vi "Sub_predictor_v4(SubVI).vi"(6 "predicted step":dbl=0.04 format="%#_13g", 8 "Sim_running":bool, 9 "q_i":dbl[](array[numeric]), 10 "Pred ?":bool, 11 "t [s]":dbl) -> (0 "Euler Angles Table [deg]":dbl[](array[numeric]), 1 "Elevation/Azimuth [deg]":dbl[](array[numeric]), 3 "Euler Angles Table_pred [deg]":dbl[](array[numeric]), 4 "DMARS SIM pred [º]":cluster{"phi":dbl, "theta":dbl, "psi":dbl})   [LabVIEW 2017]
uses:
  <vilib>/Analysis/coordinate.llb/Euler Rotation Order.ctl
  <vilib>/Analysis/_algsub.llb/Real PseudoInverse Matrix.vi
  <vilib>/Analysis/baseanly.llb/Real A x B.vi
  <vilib>/Analysis/Matrix/Numeric/Conversions/Array To Matrix - RA2.vi
  <vilib>/Analysis/Matrix/Numeric/Conversions/Array To Matrix - RA.vi
  <vilib>/Analysis/Matrix/Numeric/Conversions/Matrix To Array - RM.vi
  <vilib>/Analysis/Matrix/NI_Matrix.lvlib
  <vilib>/Analysis/NI_AALPro.lvlib
  <vilib>/Analysis/NI_AALBase.lvlib
  <vilib>/Analysis/7linalg.llb/Real Transpose Matrix.vi
panel:
  out "DCM":dbl[][](array[numeric])
  out "Elevation [deg]":dbl
  out "Azimuth [deg]":dbl
  in  "Euler Angles [º] debug":cluster{"phi":dbl, "theta":dbl, "psi":dbl}
  out "Azimuth [rad]":dbl
  out "Elevation [rad]":dbl
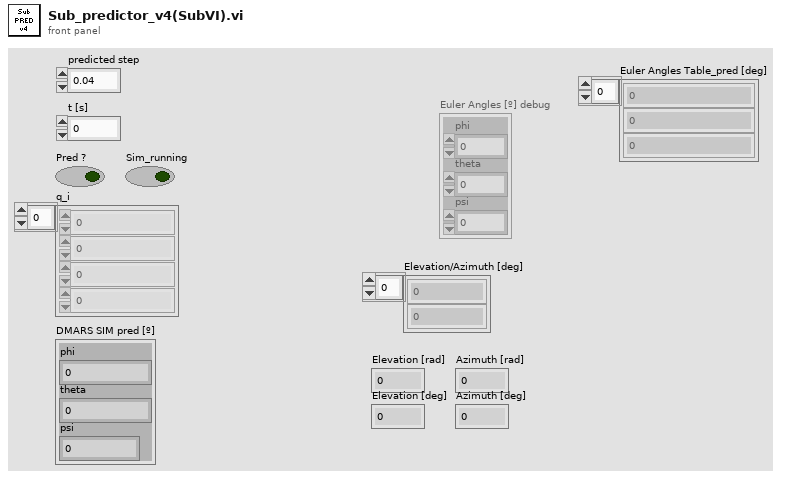
[diagram p1: front panel]
types:
  T1 = typedef "NI_Matrix.lvlib/RealMatrix.ctl" = dbl[][]
  T2 = typedef "NI_AALPro.lvlib/Euler Rotation Order.ctl" = u16
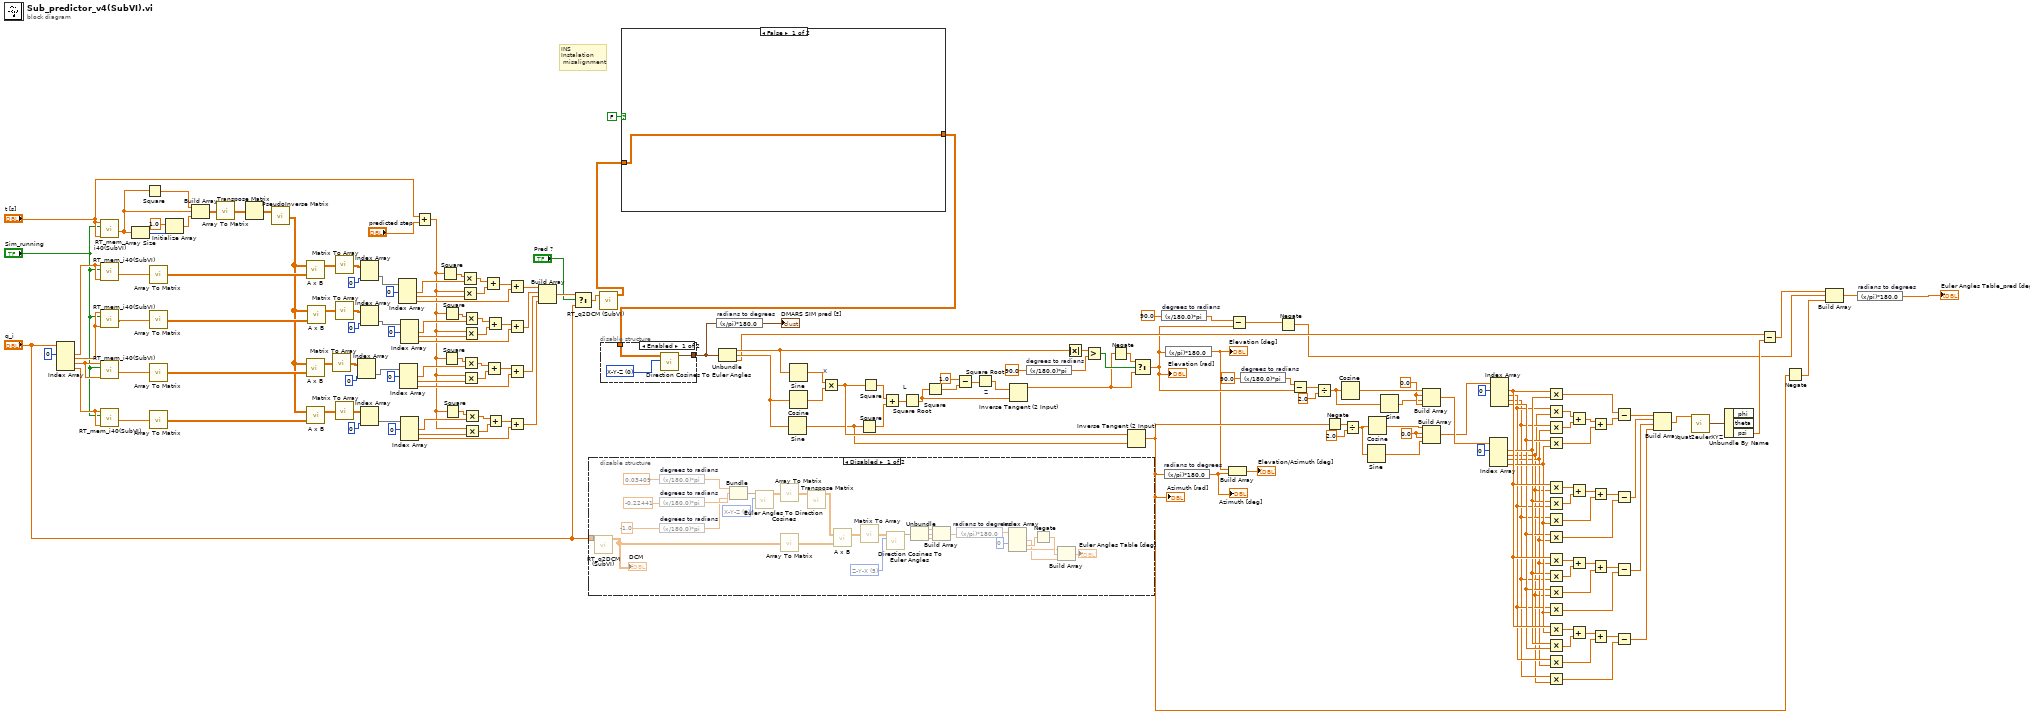
[diagram p0: block diagram]
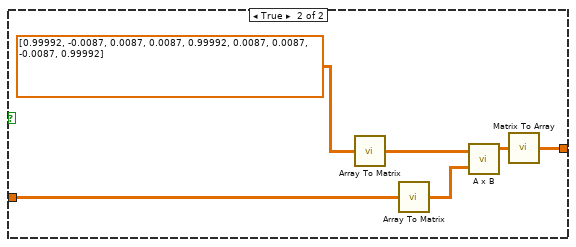
[diagram p2: hidden frame]
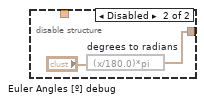
[diagram p4: hidden frame]
diagram:
  w72 = 0.0 ("element")
  w79 = 0.0 ("element")
  # "INS\nInstalation\n misalignment"
  n1 = Index Array(array="q_i", index #1=0 ("index")) -> (element #1=w101:dbl, element #2=w106:dbl, element #3=w107:dbl, element #4=w108:dbl)  [unwired: 3 in]
  n2 = call "RT_mem_i40(SubVI).vi"("Ini_val"="t [s]", "start"="Sim_running", "In"="t [s]") -> ("output array"=w109:dbl[])  [unwired: 8 in]
  n3 = call "RT_mem_i40(SubVI).vi"("Ini_val"=w101, "start"="Sim_running", "In"=w101) -> ("output array"=w104:dbl[])  [unwired: 8 in]
  n4 = call "RT_mem_i40(SubVI).vi"("Ini_val"=w106, "start"="Sim_running", "In"=w106) -> ("output array"=w105:dbl[])  [unwired: 8 in]
  n5 = call "RT_mem_i40(SubVI).vi"("Ini_val"=w107, "start"="Sim_running", "In"=w107) -> ("output array"=w103:dbl[])  [unwired: 8 in]
  n6 = call "RT_mem_i40(SubVI).vi"("Ini_val"=w108, "start"="Sim_running", "In"=w108) -> ("output array"=w102:dbl[])  [unwired: 8 in]
  n7 = Array Size(array=w109) -> (size(s)=w160:i32)
  n8 = Square(x=w109) -> (x^2=w162:dbl[])
  n9 = call-poly <vilib>:"Array To Matrix.vi"("Real 1D Array"=w104) -> ("Real Matrix (Column Vector)"=w171:T1)
  n10 = call-poly <vilib>:"Array To Matrix.vi"("Real 1D Array"=w105) -> ("Real Matrix (Column Vector)"=w167:T1)
  n11 = call-poly <vilib>:"Array To Matrix.vi"("Real 1D Array"=w103) -> ("Real Matrix (Column Vector)"=w172:T1)
  n12 = call-poly <vilib>:"Array To Matrix.vi"("Real 1D Array"=w102) -> ("Real Matrix (Column Vector)"=w159:T1)
  n13 = Initialize Array(1.0 ("element"), w160) -> (w163:dbl[])
  n14 = Build Array(w162, w109, w163) -> (w165:dbl[][])
  n15 = call-poly <vilib>:"Array To Matrix.vi"("Real 2D Array"=w165) -> ("Real Matrix"=w164:T1)
  n16 = Transpose Matrix(1:w164) -> (0:w166:T1)
  n17 = call-poly <vilib>:"PseudoInverse Matrix.vi"("Input Matrix"=w166) -> ("PseudoInverse Matrix"=w155:T1)  [unwired: 1 in, 1 out]
  n18 = call-poly <vilib>:"A x B.vi"("B"=w171, "A"=w155) -> ("A x B"=w177:T1)  [unwired: 1 out]
  n19 = call-poly <vilib>:"A x B.vi"("B"=w172, "A"=w155) -> ("A x B"=w178:T1)  [unwired: 1 out]
  n20 = call-poly <vilib>:"A x B.vi"("B"=w159, "A"=w155) -> ("A x B"=w156:T1)  [unwired: 1 out]
  n21 = call-poly <vilib>:"A x B.vi"("B"=w167, "A"=w155) -> ("A x B"=w170:T1)  [unwired: 1 out]
  n22 = call-poly <vilib>:"Matrix To Array.vi"("Real Matrix"=w178) -> ("Real 2D Array"=w175:dbl[][])
  n23 = call-poly <vilib>:"Matrix To Array.vi"("Real Matrix"=w177) -> ("Real 2D Array"=w174:dbl[][])
  n24 = call-poly <vilib>:"Matrix To Array.vi"("Real Matrix"=w170) -> ("Real 2D Array"=w168:dbl[][])
  n25 = call-poly <vilib>:"Matrix To Array.vi"("Real Matrix"=w156) -> ("Real 2D Array"=w158:dbl[][])
  n26 = Index Array(array=w175, index (col)=0 ("index (row)")) -> (element=w118:dbl[])  [unwired: 1 in]
  n27 = Index Array(array=w174, index (col)=0 ("index (row)")) -> (element=w144:dbl[])  [unwired: 1 in]
  n28 = Index Array(array=w168, index (col)=0 ("index (row)")) -> (element=w119:dbl[])  [unwired: 1 in]
  n29 = Index Array(array=w158, index (col)=0 ("index (row)")) -> (element=w117:dbl[])  [unwired: 1 in]
  n30 = Index Array(array=w144, index #1=0 ("index")) -> (element #1=w147:dbl, element #2=w149:dbl, element #3=w152:dbl)  [unwired: 2 in]
  n31 = Index Array(array=w118, index #1=0 ("index")) -> (element #1=w130:dbl, element #2=w132:dbl, element #3=w135:dbl)  [unwired: 2 in]
  n32 = Index Array(array=w119, index #1=0 ("index")) -> (element #1=w141:dbl, element #2=w139:dbl, element #3=w136:dbl)  [unwired: 2 in]
  n33 = Index Array(array=w117, index #1=0 ("index")) -> (element #1=w125:dbl, element #2=w123:dbl, element #3=w120:dbl)  [unwired: 2 in]
  n34 = Add(x="t [s]", y="predicted step") -> (x+y=w116:dbl)
  n35 = Square(x=w116) -> (x^2=w146:dbl)
  n36 = Square(x=w116) -> (x^2=w129:dbl)
  n37 = Square(x=w116) -> (x^2=w142:dbl)
  n38 = Square(x=w116) -> (x^2=w126:dbl)
  n39 = Multiply(x=w146, y=w147) -> (x*y=w148:dbl)
  n40 = Multiply(x=w116, y=w149) -> (x*y=w150:dbl)
  n41 = Multiply(x=w129, y=w130) -> (x*y=w131:dbl)
  n42 = Multiply(x=w116, y=w132) -> (x*y=w133:dbl)
  n43 = Multiply(x=w142, y=w141) -> (x*y=w140:dbl)
  n44 = Multiply(x=w116, y=w139) -> (x*y=w138:dbl)
  n45 = Multiply(x=w126, y=w125) -> (x*y=w124:dbl)
  n46 = Multiply(x=w116, y=w123) -> (x*y=w122:dbl)
  n47 = Add(x=w148, y=w150) -> (x+y=w151:dbl)
  n48 = Add(x=w131, y=w133) -> (x+y=w134:dbl)
  n49 = Add(x=w140, y=w138) -> (x+y=w137:dbl)
  n50 = Add(x=w124, y=w122) -> (x+y=w121:dbl)
  n51 = Add(x=w151, y=w152) -> (x+y=w115:dbl)
  n52 = Add(x=w137, y=w136) -> (x+y=w114:dbl)
  n53 = Add(x=w134, y=w135) -> (x+y=w113:dbl)
  n54 = Add(x=w121, y=w120) -> (x+y=w112:dbl)
  n55 = Build Array(w115, w114, w113, w112) -> (w8:dbl[])
  n56 = Select(t=w8, s="Pred ?", f="q_i") -> (s? t:f=w7:dbl[])
  n57 = disable-structure shown="Disabled" {
    disable-tunnel: "q_i" -> [w206 _]
    frame Disabled {
      w191 = T2 0 items=["X-Y-Z", "X-Z-Y", "Y-X-Z", "Y-Z-X", "Z-X-Y", "Z-Y-X", "X-Y-X", "X-Z-X", "Y-X-Y", "Y-Z-Y", "Z-X-Z", "Z-Y-Z"] ("rotation order")
      w193 = T2 5 items=["X-Y-Z", "X-Z-Y", "Y-X-Z", "Y-Z-X", "Z-X-Y", "Z-Y-X", "X-Y-X", "X-Z-X", "Y-X-Y", "Y-Z-Y", "Z-X-Z", "Z-Y-Z"] ("rotation order")
      n58 = call "RT_q2DCM (SubVI).vi"("Quaternion"=w206) -> ("DCM"=w207:dbl[][])  [unwired: 10 in]
      "DCM" <- w207
      n59 = expression code="(x/180.0)*pi" "degrees to radians"(0.03409 ("y")) -> (w190:dbl)
      n60 = expression code="(x/180.0)*pi" "degrees to radians"(-0.22441 ("y")) -> (w189:dbl)
      n61 = expression code="(x/180.0)*pi" "degrees to radians"(-1.0 ("y")) -> (w188:dbl)
      n62 = Bundle("y"=w190, "y"=w189, "y"=w188) -> (w192:cluster{"y":dbl, "y":dbl, "y":dbl})  [unwired: 1 in]
      n63 = call <vilib>:"Euler Angles To Direction Cosines.vi"("rotation order"=w191, "Euler Angles"=w192) -> ("Direction Cosines"=w185:dbl[][])  [unwired: 8 in, 1 out]
      n64 = call-poly <vilib>:"Array To Matrix.vi"("Real 2D Array"=w185) -> ("Real Matrix"=w184:T1)
      n65 = call-poly <vilib>:"Array To Matrix.vi"("Real 2D Array"=w207) -> ("Real Matrix"=w183:T1)
      n66 = call-poly <vilib>:"Transpose Matrix.vi"("Input Matrix"=w184) -> ("Matrix Transpose"=w182:T1)  [unwired: 9 in, 1 out]
      n67 = call-poly <vilib>:"A x B.vi"("B"=w183, "A"=w182) -> ("A x B"=w181:T1)  [unwired: 1 out]
      n68 = call-poly <vilib>:"Matrix To Array.vi"("Real Matrix"=w181) -> ("Real 2D Array"=w180:dbl[][])
      n69 = call <vilib>:"Direction Cosines To Euler Angles.vi"("rotation order"=w193, "Direction Cosines"=w180) -> ("Euler Angles"=w196:cluster{"phi":dbl, "theta":dbl, "psi":dbl})  [unwired: 8 in, 1 out]
      n70 = Unbundle(w196) -> ("phi"=w194:dbl, "theta"=w195:dbl, "psi"=w197:dbl)
      n71 = Build Array(w194, w195, w197) -> (w205:dbl[])
      n72 = expression code="(x/pi)*180.0" "radians to degrees"(w205) -> (w201:dbl[])
      n73 = Index Array(array=w201, index #1=0 ("index")) -> (element #1=w199:dbl, element #2=w204:dbl, element #3=w202:dbl)  [unwired: 2 in]
      n74 = Negate(x=w204) -> (-x=w203:dbl)
      n75 = Build Array(w202, w203, w199) -> (→"Euler Angles Table [deg]":dbl[])
    }
    frame Enabled {
    }
  }
  n76 = call "RT_q2DCM (SubVI).vi"("Quaternion"=w7) -> ("DCM"=w3:dbl[][])  [unwired: 10 in]
  n77 = case shown="False" FALSE {
    tunnel: [w208 w211] -> w2
    tunnel: w3 -> [w208 w209]
    frame False {
    }
    frame True {
      n78 = call-poly <vilib>:"Array To Matrix.vi"("Real 2D Array"=dbl[][] [[0.99992, -0.0087, 0.0087], [0.0087, 0.99992, 0.0087], [0.0087, -0.0087, 0.99992]]) -> ("Real Matrix"=w213:T1)
      n79 = call-poly <vilib>:"Array To Matrix.vi"("Real 2D Array"=w209) -> ("Real Matrix"=w212:T1)
      n80 = call-poly <vilib>:"A x B.vi"("B"=w212, "A"=w213) -> ("A x B"=w214:T1)  [unwired: 1 out]
      n81 = call-poly <vilib>:"Matrix To Array.vi"("Real Matrix"=w214) -> ("Real 2D Array"=w211:dbl[][])
    }
  }
  n82 = disable-structure shown="Enabled" {
    disable-tunnel: [w217 w218] -> w15
    disable-tunnel: w2 -> [w215 _]
    frame Enabled {
      w216 = T2 0 items=["X-Y-Z", "X-Z-Y", "Y-X-Z", "Y-Z-X", "Z-X-Y", "Z-Y-X", "X-Y-X", "X-Z-X", "Y-X-Y", "Y-Z-Y", "Z-X-Z", "Z-Y-Z"] ("rotation order")
      n83 = call <vilib>:"Direction Cosines To Euler Angles.vi"("rotation order"=w216, "Direction Cosines"=w215) -> ("Euler Angles"=w217:cluster{"phi":dbl, "theta":dbl, "psi":dbl})  [unwired: 8 in, 1 out]
    }
    frame Disabled {
      n84 = expression code="(x/180.0)*pi" "degrees to radians"("Euler Angles [º] debug") -> (w218:cluster{"phi":dbl, "theta":dbl, "psi":dbl})
    }
  }
  n85 = expression code="(x/pi)*180.0" "radians to degrees"(w15) -> (→"DMARS SIM pred [º]":cluster{"phi":dbl, "theta":dbl, "psi":dbl})
  n86 = Unbundle(w15) -> ("phi"=w89:dbl, "theta"=w97:dbl, "psi"=w28:dbl)
  n87 = Sine(x=w97) -> (sin(x)=w82:dbl)
  n88 = Sine(x=w89) -> (sin(x)=w99:dbl)
  n89 = Cosine(x=w97) -> (cos(x)=w98:dbl)
  n90 = Multiply "X"(x=w99, y=w98) -> (x*y=w83:dbl)
  n91 = Square(x=w82) -> (x^2=w95:dbl)
  n92 = Square(x=w83) -> (x^2=w96:dbl)
  n93 = Add(x=w96, y=w95) -> (x+y=w94:dbl)
  n94 = Square Root "L"(x=w94) -> (sqrt(x)=w91:dbl)
  n95 = Square(x=w91) -> (x^2=w93:dbl)
  n96 = Subtract(x=1.0, y=w93) -> (x-y=w17:dbl)
  n97 = Square Root "Z"(x=w17) -> (sqrt(x)=w16:dbl)
  n98 = Inverse Tangent (2 Input)(1:w91, 2:w16) -> (0:w84:dbl)
  n99 = expression code="(x/180.0)*pi" "degrees to radians"(90.0 ("y")) -> (w87:dbl)
  n100 = Absolute Value(x=w89) -> (abs(x)=w88:dbl)
  n101 = Greater?(x=w88, y=w87) -> (0:w86:bool)
  n102 = Negate(x=w84) -> (-x=w85:dbl)
  n103 = Inverse Tangent (2 Input)(1:w82, 2:w83) -> (0:w13:dbl)
  "Azimuth [rad]" <- w13
  n104 = Select(t=w85, s=w86, f=w84) -> (s? t:f=w12:dbl)
  "Elevation [rad]" <- w12
  n105 = expression code="(x/180.0)*pi" "degrees to radians"(90.0 ("y")) -> (w20:dbl)
  n106 = expression code="(x/pi)*180.0" "radians to degrees"(w13) -> (w10:dbl)
  "Azimuth [deg]" <- w10
  n107 = expression code="(x/pi)*180.0" ("radians to degrees")(w12) -> (w11:dbl)
  "Elevation [deg]" <- w11
  n108 = Build Array(w11, w10) -> (→"Elevation/Azimuth [deg]":dbl[])
  n109 = Subtract(x=w20, y=w12) -> (x-y=w19:dbl)
  n110 = expression code="(x/180.0)*pi" "degrees to radians"(90.0 ("y")) -> (w75:dbl)
  n111 = Negate(x=w19) -> (-x=w18:dbl)
  n112 = Subtract(x=w75, y=w12) -> (x-y=w25:dbl)
  n113 = Divide(x=w25, y=2.0) -> (x/y=w70:dbl)
  n114 = Negate(x=w13) -> (-x=w81:dbl)
  n115 = Cosine(x=w70) -> (cos(x)=w73:dbl)
  n116 = Divide(x=w81, y=2.0) -> (x/y=w78:dbl)
  n117 = Sine(x=w78) -> (sin(x)=w77:dbl)
  n118 = Cosine(x=w78) -> (cos(x)=w71:dbl)
  n119 = Sine(x=w70) -> (sin(x)=w69:dbl)
  n120 = Build Array(w73, w72, w69, w72) -> (w23:dbl[])
  n121 = Build Array(w71, w79, w79, w77) -> (w22:dbl[])
  n122 = Index Array(array=w23, index #1=0 ("index")) -> (element #1=w37:dbl, element #2=w32:dbl, element #3=w34:dbl, element #4=w38:dbl)  [unwired: 3 in]
  n123 = Index Array(array=w22, index #1=0 ("index")) -> (element #1=w39:dbl, element #2=w35:dbl, element #3=w33:dbl, element #4=w36:dbl)  [unwired: 3 in]
  n124 = Multiply(x=w39, y=w37) -> (x*y=w61:dbl)
  n125 = Multiply(x=w35, y=w32) -> (x*y=w66:dbl)
  n126 = Multiply(x=w33, y=w34) -> (x*y=w65:dbl)
  n127 = Multiply(x=w36, y=w38) -> (x*y=w63:dbl)
  n128 = Multiply(x=w39, y=w32) -> (x*y=w59:dbl)
  n129 = Multiply(x=w37, y=w35) -> (x*y=w58:dbl)
  n130 = Multiply(x=w33, y=w38) -> (x*y=w55:dbl)
  n131 = Multiply(x=w36, y=w34) -> (x*y=w54:dbl)
  n132 = Multiply(x=w39, y=w34) -> (x*y=w47:dbl)
  n133 = Multiply(x=w37, y=w33) -> (x*y=w48:dbl)
  n134 = Multiply(x=w36, y=w32) -> (x*y=w51:dbl)
  n135 = Multiply(x=w35, y=w38) -> (x*y=w52:dbl)
  n136 = Multiply(x=w39, y=w38) -> (x*y=w45:dbl)
  n137 = Multiply(x=w37, y=w36) -> (x*y=w44:dbl)
  n138 = Multiply(x=w35, y=w34) -> (x*y=w41:dbl)
  n139 = Multiply(x=w33, y=w32) -> (x*y=w40:dbl)
  n140 = Add(x=w66, y=w65) -> (x+y=w64:dbl)
  n141 = Add(x=w59, y=w58) -> (x+y=w57:dbl)
  n142 = Add(x=w47, y=w48) -> (x+y=w49:dbl)
  n143 = Add(x=w45, y=w44) -> (x+y=w43:dbl)
  n144 = Add(x=w64, y=w63) -> (x+y=w62:dbl)
  n145 = Add(x=w57, y=w55) -> (x+y=w56:dbl)
  n146 = Add(x=w49, y=w51) -> (x+y=w50:dbl)
  n147 = Add(x=w43, y=w41) -> (x+y=w42:dbl)
  n148 = Subtract(x=w61, y=w62) -> (x-y=w60:dbl)
  n149 = Subtract(x=w56, y=w54) -> (x-y=w53:dbl)
  n150 = Subtract(x=w50, y=w52) -> (x-y=w46:dbl)
  n151 = Subtract(x=w42, y=w40) -> (x-y=w31:dbl)
  n152 = Build Array(w60, w53, w46, w31) -> (w30:dbl[])
  n153 = call "quat2eulerXYZ.vi"("Quaternions"=w30) -> ("Euler Angles [rad]"=w29:cluster{"phi":dbl, "theta":dbl, "psi":dbl})  [unwired: 10 in]
  n154 = Unbundle By Name(w29) -> ("psi"=w27:dbl)  [unwired: 2 out]
  n155 = Subtract(x=w28, y=w27) -> (x-y=w26:dbl)
  n156 = Negate(x=w13) -> (-x=w24:dbl)
  n157 = Build Array(w26, w18, w24) -> (w1:dbl[])
  n158 = expression code="(x/pi)*180.0" "radians to degrees"(w1) -> (→"Euler Angles Table_pred [deg]":dbl[])
